vi "delta.vi"() -> (3 "Array":dbl[](array[numeric]))   [LabVIEW 2020]
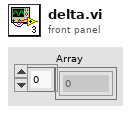
[diagram p1: front panel]
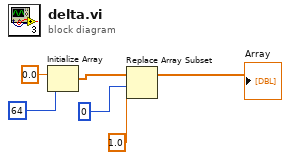
[diagram p0: block diagram]
diagram:
  n1 = Initialize Array(0.0 ("element"), 64 ("dimension size")) -> (w3:dbl[])
  n2 = Replace Array Subset(array=w3, new element=1.0 ("new element/subarray"), index=0) -> (→"Array":dbl[])
